vi "States.vi"(8 "error in (no error)":errorcluster, 11 "Sequence Config in":refnum<class "Sequence Config.lvclass">) -> (0 "error out":errorcluster, 2 "States":map{string, T1}(c390), 3 "Sequence Config out":refnum<class "Sequence Config.lvclass">)   [LabVIEW 2020, in "VolatusSeqConfig.lvlib" / "Sequence Config.lvclass"]
uses:
  Sequence Config.lvclass
  Sequence Config.lvclass/Sequence Config.ctl
  Command Config/Command Config.lvclass
  Step.ctl
  VolatusSeqConfig.lvlib
  Transition Config/Transition Config.lvclass
  State.ctl
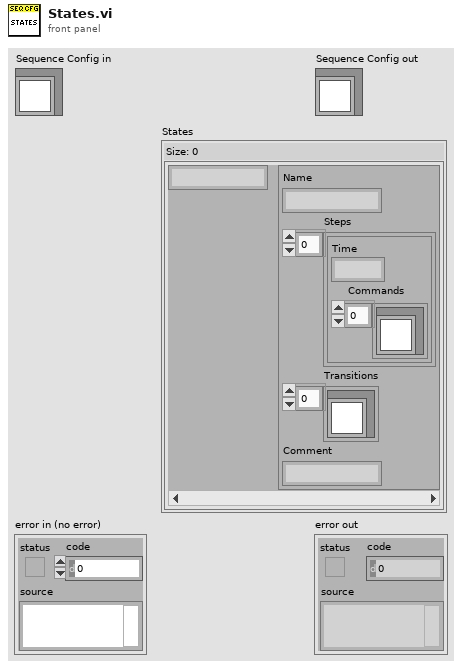
[diagram p1: front panel]
types:
  T1 = typedef "VolatusSeqConfig.lvlib/State.ctl" = cluster{"Name":string, "Steps":T2[], "Transitions":refnum<class "Transition Config.lvclass">[], "Comment":string}
  T2 = typedef "VolatusSeqConfig.lvlib/Step.ctl" = cluster{"Time":dbl, "Commands":refnum<class "Command Config.lvclass">[]}
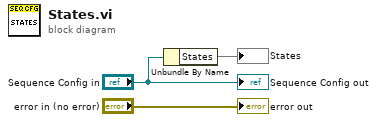
[diagram p0: block diagram]
diagram:
  n1 = Unbundle By Name("Sequence Config in") -> ("States"=→"States":map{string, T1})
  "error out" <- "error in (no error)"
  "Sequence Config out" <- "Sequence Config in"
